vi "appendScanFor LogMaker.vi"(8 "error in (no error)":errorcluster, 11 "New Google\nExpLog for new day?":bool) -> (3 "standard output":string)   [LabVIEW 2020]
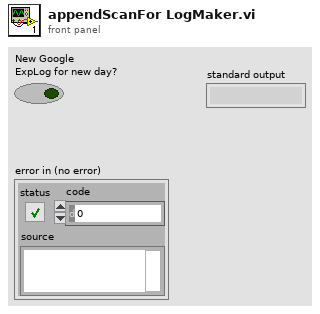
[diagram p1: front panel]
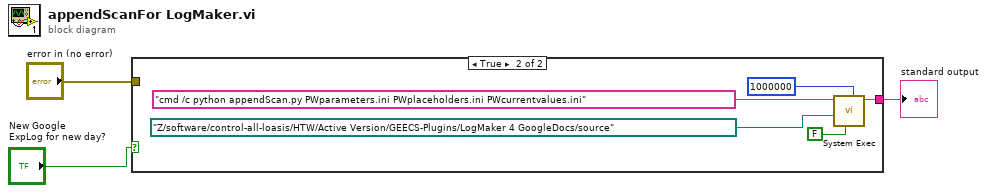
[diagram p0: block diagram]
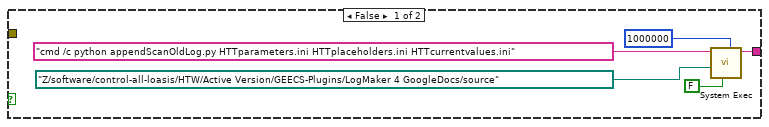
[diagram p2: hidden frame]
diagram:
  n1 = case shown="True" "New Google\nExpLog for new day?" {
    tunnel: [w4 w9] -> w2
    tunnel: "error in (no error)" -> [_ _]
    frame False {
      n2 = call <vilib>:"System Exec.vi"("expected output size  (4096)"=u32 1000000, "run minimized? (F)"=FALSE, "working directory"=path "Z:/software/control-all-loasis/HTW/Active Version/GEECS-Plugins/LogMaker 4 GoogleDocs/source", "command line"="cmd /c python appendScanOldLog.py HTTparameters.ini HTTplaceholders.ini HTTcurrentvalues.ini") -> ("standard output"=w4:string)  [unwired: 4 in, 3 out]
    }
    frame True {
      n3 = call <vilib>:"System Exec.vi"("expected output size  (4096)"=u32 1000000, "run minimized? (F)"=FALSE, "working directory"=path "Z:/software/control-all-loasis/HTW/Active Version/GEECS-Plugins/LogMaker 4 GoogleDocs/source", "command line"="cmd /c python appendScan.py PWparameters.ini PWplaceholders.ini PWcurrentvalues.ini") -> ("standard output"=w9:string)  [unwired: 4 in, 3 out]
    }
  }
  "standard output" <- w2
